vi "SVL Running Leq Sound Level (N Ch).vi"(6 "restart averaging (F)":bool, 8 "error in (no error)":errorcluster, 9 "integration time [s]":dbl=1.0 format="%.2f", 11 "scaled signals [EU]":waveform(dbl)[](array[waveform])) -> (0 "error out":errorcluster, 1 "actual integration time [s]":dbl=nan format="%.2f", 2 "unit labels":string[](array[string]), 3 "running Leq sound levels [dB EU]":dbl[](array[numeric]) format="%.2f")   [LabVIEW 2017, in "SoundVib_SoundLevel.lvlib"]
doc: "Computes the running equivalent continuous sound level (Leq) of <B>scaled signal [EU]</B>. <B>scaled signal [EU]</B> should have a zero DC component. Wire data to the <B>scaled signal [EU]</B> input to determine the polymorphic instance to use or manually select the instance."
uses:
  <vilib>/addons/Sound and Vibration/svt_Level/SoundVib_SoundLevel.lvlib
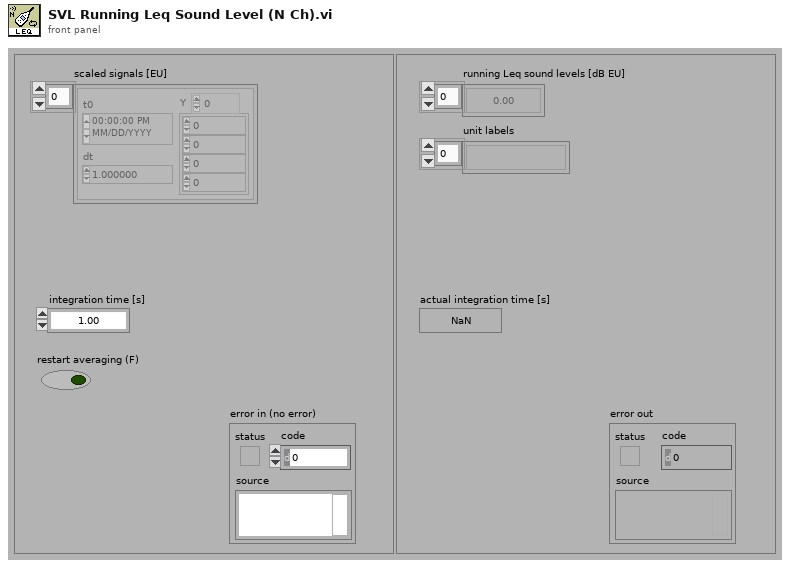
[diagram p1: front panel]
types:
  T1 = enum16{"RMS", "Running RMS", "Exp avg  ", "Dec exp avg ", "Peak", "Crest"}
  T2 = enum16{"Reset filter", "Restart averaging", "Continue processing"}
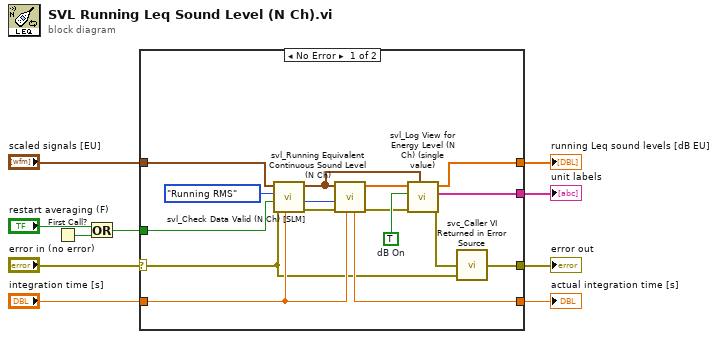
[diagram p0: block diagram]
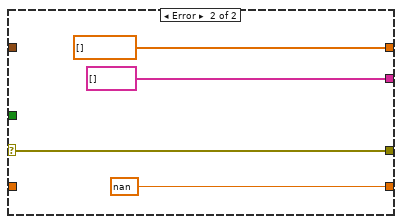
[diagram p2: hidden frame]
diagram:
  n1 = First Call?() -> (First Call?: T/F=w5:bool)
  n2 = Or(x="restart averaging (F)", y=w5) -> (x .or. y?=w2:bool)
  n3 = case shown="No Error" "error in (no error)" {
    selector: "error in (no error)" -> [w11 w30]
    tunnel: [w26 dbl[] [] ("energy levels [EU^2 rms]")] -> w10
    tunnel: [w25 string[] [] ("unit label [ ]")] -> w9
    tunnel: [w20 w30] -> w8
    tunnel: [w19 nan ("actual integration time [s]")] -> w7
    tunnel: "integration time [s]" -> [w15 _]
    tunnel: "scaled signals [EU]" -> [w12 _]
    tunnel: w2 -> [w16 _]
    frame No Error {
      w23 = TRUE  # dB On
      n4 = call <vilib>:"svl_Check Data Valid (N Ch) [SLM].vi"("integration time [s]"=w15, "error in (no error)"=w11, "restart averaging (F)"=w16, "level analysis"=T1."Running RMS" ("Level Analysis"), "scaled signals [EU]"=w12) -> ("error out"=w18:errorcluster, "processing state"=w17:T2, "dup scaled signals [EU]"=w13:waveform(dbl)[])  [unwired: 4 in]
      n5 = call <vilib>:"svl_Running Equivalent Continuous Sound Level (N Ch).vi"("integration time [s]"=w15, "error in (no error)"=w18, "processing state"=w17, "scaled signals [EU]"=w13) -> ("error out"=w21:errorcluster, "energy level [ ] [EU^2 rms]"=w22:dbl[], "actual integration time [s]"=w19:dbl)  [unwired: 5 in]
      n6 = call <vilib>:"svl_Log View for Energy Level (N Ch) (single value).vi"("waveform parameters"=w13, "error in (no error)"=w21, "dB On (T)"=w23, "energy levels [EU^2 rms]"=w22) -> ("error out"=w24:errorcluster, "unit label [ ]"=w25:string[], "energy levels [EU^2 rms]"=w26:dbl[])  [unwired: 5 in]
      n7 = call <vilib>:"svc_Caller VI Returned in Error Source.vi"("warning input to caller"=w11, "error in (no error)"=w24) -> ("error out"=w20:errorcluster)  [unwired: 3 in]
    }
    frame Error {
    }
  }
  "running Leq sound levels [dB EU]" <- w10
  "unit labels" <- w9
  "error out" <- w8
  "actual integration time [s]" <- w7
